vi "SIM Registry Report Registry Error.vi"(9 "code":i32, 10 "Block Idx":i32, 11 "Registry Error":T1) -> (3 "Registry Error Out":T1)   [LabVIEW 2017]
uses:
  <vilib>/Simulation/Implementation/Shared/SIM Registry.llb/SIM Simulation Registry Error.ctl
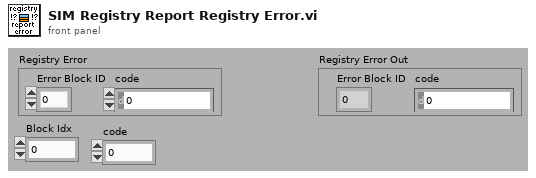
[diagram p1: front panel]
types:
  T1 = typedef "SIM Simulation Registry Error.ctl" = cluster{"Error Block ID":i32, "code":i32}
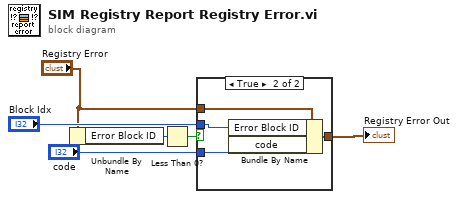
[diagram p0: block diagram]
diagram:
  n1 = Unbundle By Name("Registry Error") -> ("Error Block ID"=w1:i32)
  n2 = Less Than 0?(x=w1) -> (x < 0?=w2:bool)
  n3 = case shown="True" w2 {
    tunnel: "Registry Error" -> [w7 w11]
    tunnel: [w7 w10] -> w4
    tunnel: "Block Idx" -> [_ w9]
    tunnel: "code" -> [_ w8]
    frame False {
    }
    frame True {
      n4 = Bundle By Name(cluster=w11, "Error Block ID"=w9, "code"=w8) -> (w10:T1)
    }
  }
  "Registry Error Out" <- w4
